vi "1_VisualAD_Train_Eval.vi"(0 "NNFE_Paths":T11={"CFG"=path "D:/Ngene/Projects_SVN/AD/Models/0_Orig/WRN_50_2_1/WRN_50_2_1.cfg", "BIN"=path "D:/Ngene/Projects_SVN/AD/Models/0_Orig/WRN_50_2_1/WRN_50_2_1.bin"}, 1 "Dest. Path":path=path "D:/working/PCB5_append_2025_04_21/21_Data_Leak_Cleaned", 2 "Dataset_Path(Train)":path=path "D:/DNN/_from_Customer/2025_04_11_NIConnect_PCB5/1_Dataset/21_Data_Leak/Train", 3 "Dataset_Path(Validation)":path=path "D:/DNN/_from_Customer/2025_04_11_NIConnect_PCB5/1_Dataset/21_Data_Leak/Test", 4 "Ground_Truth_Folder_Path":path, 5 "error in":errorcluster, 6 "NNFE_CFG":T7={"Name"="PCB5_10K", "Layer_Selection_By"=enum."Stride", "Feature_Layers"={"[LayerID, PatchSize]"=[{"Layer_ID"=8, "Patch_Size"=3}, {"Layer_ID"=16, "Patch_Size"=3}]}, "Interpolation_Type"=enum."Bi-Linear"}, 7 "Dim_Reduction":T5={"Method"=enum."Rnd_Proj", "Target_Dim"=300, "Seed"=42}, 8 "NNPC_Setup":T13={"Input_Dims"={"C"=3, "H"=464, "W"=464}, "mBatch"=1, "Device"=enum."GPU", "GPU Id"=0}, 9 "Coreset_Params":T12={"CoreSet_Size"=10000.0, "Start_idx"=3}) -> (11 "MemBank Size":i32=10000, 13 "dT_Total":dbl=154.27649250000002 format="%.2p", 14 "NNPC_Paths":T11={"CFG"=path "D:/working/PCB5_append_2025_04_21/21_Data_Leak_Cleaned/NNPC_PCB5_10K__25_04_24__18_51_48/NNPC_PCB5_10K.cfg", "BIN"=path "D:/working/PCB5_append_2025_04_21/21_Data_Leak_Cleaned/NNPC_PCB5_10K__25_04_24__18_51_48/NNPC_PCB5_10K.bin"}, 15 "Evaluation_Metrics":T1={"Evaluation_Metrics(Pixel)"={"Scores(Good)"={"X Values"=[0.1535603703558445, 0.16897603914141654, 0.1843917079269886, 0.19980737671256066, 0.2152230454981327, 0.23063871428370475, 0.24605438306927682, 0.26147005185484884, 0.27688572064042094, 0.29230138942599293, 0.30771705821156503, 0.3231327269971371, 0.3385483957827091, 0.35396406456828117, 0.3693797333538532, 0.3847954021394253, 0.4002110709249973, 0.4156267397105694, 0.4310424084961414, 0.4464580772817135, 0.46187374606728554, 0.4772894148528576, 0.4927050836384297, 0.5081207524240017, 0.5235364212095738, 0.5389520899951458, 0.5543677587807179, 0.5697834275662899, 0.585199096351862, 0.6006147651374341, 0.616030433923006, 0.6314461027085781, 0.6468617714941503, 0.6622774402797222, 0.6776931090652942, 0.6931087778508663, 0.7085244466364384, 0.7239401154220104, 0.7393557842075824, 0.7547714529931545, 0.7701871217787266, 0.7856027905642986, 0.8010184593498707, 0.8164341281354428, 0.8318497969210148, 0.8472654657065868, 0.8626811344921589, 0.878096803277731, 0.893512472063303, 0.9089281408488751, 0.9243438096344472, 0.9397594784200192, 0.9551751472055912, 0.9705908159911633, 0.9860064847767354, 1.0014221535623073, 1.0168378223478793, 1.0322534911334516, 1.0476691599190235, 1.0630848287045955, 1.0785004974901677, 1.0939161662757397, 1.1093318350613117, 1.1247475038468837, 1.1401631726324557, 1.155578841418028, 1.1709945102036001, 1.186410178989172, 1.201825847774744, 1.217241516560316, 1.232657185345888, 1.2480728541314603, 1.2634885229170323, 1.2789041917026043, 1.2943198604881765, 1.3097355292737483, 1.3251511980593205, 1.3405668668448927, 1.3559825356304644, 1.3713982044160367, 1.3868138732016086, 1.4022295419871806, 1.4176452107727529, 1.4330608795583248, 1.4484765483438968, 1.463892217129469, 1.4793078859150408, 1.494723554700613, 1.5101392234861852, 1.525554892271757, 1.5409705610573292, 1.5563862298429014, 1.5718018986284732, 1.5872175674140454, 1.6026332361996174, 1.6180489049851894, 1.6334645737707616, 1.6488802425563336, 1.6642959113419056, 1.6797115801274778], "Histogram: h(x)"=[19, 71, 234, 537, 635, 791, 1187, 1664, 4455, 11669, 20450, 27156, 34487, 49909, 89115, 129180, 121277, 93394, 90513, 113616, 128442, 115986, 110386, 119416, 134560, 135091, 138673, 148501, 164573, 180077, 199799, 237706, 287334, 355240, 447708, 578830, 783339, 1110851, 1567027, 2139067, 2671026, 3035938, 3160582, 3051610, 2749404, 2402005, 2090427, 1813597, 1650279, 1570001, 1566516, 1637595, 1767667, 1922699, 2103025, 2248584, 2331421, 2335270, 2221028, 1978020, 1626686, 1226441, 847834, 527127, 293111, 152894, 74763, 33902, 15905, 7259, 3291, 1305, 482, 241, 145, 57, 2, 0, 0, 0, 0, 0, 0, 0, 0, 0, 0, 0, 0, 0, 0, 0, 0, 0, 0, 0, 0, 0, 0, 0]}, "Scores(Bad)"={"X Values"=[0.1535603703558445, 0.16897603914141654, 0.1843917079269886, 0.19980737671256066, 0.2152230454981327, 0.23063871428370475, 0.24605438306927682, 0.26147005185484884, 0.27688572064042094, 0.29230138942599293, 0.30771705821156503, 0.3231327269971371, 0.3385483957827091, 0.35396406456828117, 0.3693797333538532, 0.3847954021394253, 0.4002110709249973, 0.4156267397105694, 0.4310424084961414, 0.4464580772817135, 0.46187374606728554, 0.4772894148528576, 0.4927050836384297, 0.5081207524240017, 0.5235364212095738, 0.5389520899951458, 0.5543677587807179, 0.5697834275662899, 0.585199096351862, 0.6006147651374341, 0.616030433923006, 0.6314461027085781, 0.6468617714941503, 0.6622774402797222, 0.6776931090652942, 0.6931087778508663, 0.7085244466364384, 0.7239401154220104, 0.7393557842075824, 0.7547714529931545, 0.7701871217787266, 0.7856027905642986, 0.8010184593498707, 0.8164341281354428, 0.8318497969210148, 0.8472654657065868, 0.8626811344921589, 0.878096803277731, 0.893512472063303, 0.9089281408488751, 0.9243438096344472, 0.9397594784200192, 0.9551751472055912, 0.9705908159911633, 0.9860064847767354, 1.0014221535623073, 1.0168378223478793, 1.0322534911334516, 1.0476691599190235, 1.0630848287045955, 1.0785004974901677, 1.0939161662757397, 1.1093318350613117, 1.1247475038468837, 1.1401631726324557, 1.155578841418028, 1.1709945102036001, 1.186410178989172, 1.201825847774744, 1.217241516560316, 1.232657185345888, 1.2480728541314603, 1.2634885229170323, 1.2789041917026043, 1.2943198604881765, 1.3097355292737483, 1.3251511980593205, 1.3405668668448927, 1.3559825356304644, 1.3713982044160367, 1.3868138732016086, 1.4022295419871806, 1.4176452107727529, 1.4330608795583248, 1.4484765483438968, 1.463892217129469, 1.4793078859150408, 1.494723554700613, 1.5101392234861852, 1.525554892271757, 1.5409705610573292, 1.5563862298429014, 1.5718018986284732, 1.5872175674140454, 1.6026332361996174, 1.6180489049851894, 1.6334645737707616, 1.6488802425563336, 1.6642959113419056, 1.6797115801274778], "Histogram: h(x)"=[15, 62, 167, 436, 439, 636, 953, 1430, 4212, 9790, 18668, 24642, 27931, 41152, 76605, 105284, 87120, 64040, 68221, 91456, 99939, 85338, 81368, 91950, 104560, 104089, 104569, 115887, 129349, 141297, 162320, 197756, 245867, 310594, 398093, 521655, 715567, 1011400, 1434978, 1933150, 2371176, 2625090, 2582296, 2318639, 1934602, 1521878, 1169314, 929512, 776429, 692764, 672584, 701745, 761058, 844568, 931450, 1018644, 1115656, 1203961, 1254942, 1264724, 1221327, 1119570, 973888, 796667, 632049, 490256, 379906, 296566, 239752, 201233, 178240, 157317, 141343, 130655, 120745, 108950, 97346, 86684, 74229, 61719, 51335, 41546, 34304, 27697, 21602, 18168, 14874, 11980, 8282, 5622, 4047, 3122, 1867, 1094, 601, 280, 136, 86, 64, 34]}, "Eval Stats"={"Scores(Good)"={"Min"=0.14585254, "Max"=1.317711}, "Scores(Bad)"={"Min"=0.15503743, "Max"=1.6874194}, "# of Samples(Good)"=58991104, "# of Samples(Bad)"=43059200, "AUROC"=0.5022648, "F1_Max"=0.5934719, "Thrshld(F1_Max)"=0.1551112, "Prec.(F1_Max)"=0.42194095, "Recall(F1_Max)"=1.0, "FPR(F1_Max)"=0.9999999, "FNR(F1_Max)"=2.322384e-08}}, "Evaluation_Metrics(Image)"={"Scores(Good)"={"X Values"=[1.0789142006635666, 1.0860141378641128, 1.093114075064659, 1.1002140122652053, 1.1073139494657516, 1.1144138866662978, 1.1215138238668443, 1.1286137610673905, 1.1357136982679368, 1.142813635468483, 1.1499135726690293, 1.1570135098695755, 1.1641134470701218, 1.171213384270668, 1.1783133214712143, 1.1854132586717605, 1.1925131958723068, 1.199613133072853, 1.2067130702733992, 1.2138130074739457, 1.220912944674492, 1.2280128818750382, 1.2351128190755845, 1.2422127562761307, 1.249312693476677, 1.2564126306772232, 1.2635125678777694, 1.2706125050783157, 1.277712442278862, 1.2848123794794082, 1.2919123166799544, 1.2990122538805007, 1.3061121910810471, 1.3132121282815934, 1.3203120654821396, 1.3274120026826859, 1.3345119398832321, 1.3416118770837784, 1.3487118142843246, 1.3558117514848709, 1.3629116886854171, 1.3700116258859634, 1.3771115630865096, 1.3842115002870559, 1.3913114374876023, 1.3984113746881486, 1.4055113118886948, 1.412611249089241, 1.4197111862897873, 1.4268111234903336, 1.4339110606908798, 1.441010997891426, 1.4481109350919723, 1.4552108722925186, 1.4623108094930648, 1.469410746693611, 1.4765106838941573, 1.4836106210947035, 1.4907105582952498, 1.4978104954957963, 1.5049104326963425, 1.5120103698968888, 1.519110307097435, 1.5262102442979812, 1.5333101814985275, 1.5404101186990737, 1.54751005589962, 1.5546099931001662, 1.5617099303007125, 1.568809867501259, 1.5759098047018052, 1.5830097419023514, 1.5901096791028977, 1.597209616303444, 1.6043095535039902, 1.6114094907045364, 1.6185094279050827, 1.625609365105629, 1.6327093023061752, 1.6398092395067214, 1.6469091767072677, 1.654009113907814, 1.6611090511083602, 1.6682089883089064, 1.6753089255094527, 1.682408862709999, 1.6895087999105454, 1.6966087371110916, 1.7037086743116379, 1.710808611512184, 1.7179085487127304, 1.7250084859132766, 1.7321084231138228, 1.7392083603143693, 1.7463082975149156, 1.7534082347154618, 1.760508171916008, 1.7676081091165543, 1.7747080463171006, 1.7818079835176468], "Histogram: h(x)"=[1, 0, 0, 0, 0, 0, 0, 0, 0, 0, 0, 1, 0, 0, 0, 0, 1, 2, 2, 4, 7, 21, 16, 24, 30, 12, 19, 17, 23, 18, 11, 7, 9, 7, 14, 6, 2, 6, 5, 1, 3, 0, 0, 1, 1, 1, 0, 1, 0, 1, 0, 0, 0, 0, 0, 0, 0, 0, 0, 0, 0, 0, 0, 0, 0, 0, 0, 0, 0, 0, 0, 0, 0, 0, 0, 0, 0, 0, 0, 0, 0, 0, 0, 0, 0, 0, 0, 0, 0, 0, 0, 0, 0, 0, 0, 0, 0, 0, 0, 0]}, "Scores(Bad)"={"X Values"=[1.0789142006635666, 1.0860141378641128, 1.093114075064659, 1.1002140122652053, 1.1073139494657516, 1.1144138866662978, 1.1215138238668443, 1.1286137610673905, 1.1357136982679368, 1.142813635468483, 1.1499135726690293, 1.1570135098695755, 1.1641134470701218, 1.171213384270668, 1.1783133214712143, 1.1854132586717605, 1.1925131958723068, 1.199613133072853, 1.2067130702733992, 1.2138130074739457, 1.220912944674492, 1.2280128818750382, 1.2351128190755845, 1.2422127562761307, 1.249312693476677, 1.2564126306772232, 1.2635125678777694, 1.2706125050783157, 1.277712442278862, 1.2848123794794082, 1.2919123166799544, 1.2990122538805007, 1.3061121910810471, 1.3132121282815934, 1.3203120654821396, 1.3274120026826859, 1.3345119398832321, 1.3416118770837784, 1.3487118142843246, 1.3558117514848709, 1.3629116886854171, 1.3700116258859634, 1.3771115630865096, 1.3842115002870559, 1.3913114374876023, 1.3984113746881486, 1.4055113118886948, 1.412611249089241, 1.4197111862897873, 1.4268111234903336, 1.4339110606908798, 1.441010997891426, 1.4481109350919723, 1.4552108722925186, 1.4623108094930648, 1.469410746693611, 1.4765106838941573, 1.4836106210947035, 1.4907105582952498, 1.4978104954957963, 1.5049104326963425, 1.5120103698968888, 1.519110307097435, 1.5262102442979812, 1.5333101814985275, 1.5404101186990737, 1.54751005589962, 1.5546099931001662, 1.5617099303007125, 1.568809867501259, 1.5759098047018052, 1.5830097419023514, 1.5901096791028977, 1.597209616303444, 1.6043095535039902, 1.6114094907045364, 1.6185094279050827, 1.625609365105629, 1.6327093023061752, 1.6398092395067214, 1.6469091767072677, 1.654009113907814, 1.6611090511083602, 1.6682089883089064, 1.6753089255094527, 1.682408862709999, 1.6895087999105454, 1.6966087371110916, 1.7037086743116379, 1.710808611512184, 1.7179085487127304, 1.7250084859132766, 1.7321084231138228, 1.7392083603143693, 1.7463082975149156, 1.7534082347154618, 1.760508171916008, 1.7676081091165543, 1.7747080463171006, 1.7818079835176468], "Histogram: h(x)"=[0, 0, 0, 0, 0, 0, 0, 0, 0, 0, 0, 0, 0, 0, 0, 0, 0, 0, 0, 0, 0, 0, 0, 0, 0, 0, 0, 0, 0, 0, 0, 0, 0, 0, 0, 0, 0, 0, 0, 0, 0, 0, 0, 0, 0, 0, 0, 0, 0, 0, 0, 0, 0, 1, 0, 0, 1, 1, 2, 1, 6, 1, 3, 10, 5, 5, 7, 5, 15, 17, 9, 11, 13, 7, 10, 10, 8, 7, 6, 4, 7, 5, 7, 3, 4, 3, 3, 1, 0, 1, 0, 0, 0, 0, 0, 0, 0, 0, 0, 1]}, "Eval Stats"={"Scores(Good)"={"Min"=1.0753642, "Max"=1.4269079}, "Scores(Bad)"={"Min"=1.4559232, "Max"=1.785358}, "# of Samples(Good)"=274, "# of Samples(Bad)"=200, "AUROC"=1.0, "F1_Max"=1.0, "Thrshld(F1_Max)"=1.4414155, "Prec.(F1_Max)"=1.0, "Recall(F1_Max)"=1.0, "FPR(F1_Max)"=0.0, "FNR(F1_Max)"=0.0}}} {"Evaluation_Metrics(Image)"."Eval Stats"."Recall(F1_Max)" format="%#.5f"; "Evaluation_Metrics(Image)"."Eval Stats"."FPR(F1_Max)" format="%#.5f"; "Evaluation_Metrics(Image)"."Eval Stats"."FNR(F1_Max)" format="%#.5f"; "Evaluation_Metrics(Image)"."Eval Stats"."Prec.(F1_Max)" format="%#.5f"; "Evaluation_Metrics(Image)"."Eval Stats"."F1_Max" format="%#.5f"; "Evaluation_Metrics(Image)"."Eval Stats"."AUROC" format="%#.5f"; "Evaluation_Metrics(Image)"."Eval Stats"."Scores(Bad)"."Min" format="%#_5g"; "Evaluation_Metrics(Image)"."Eval Stats"."Scores(Good)"."Min" format="%#_5g"; "Evaluation_Metrics(Image)"."Eval Stats"."Thrshld(F1_Max)" format="%#_5f"; "Evaluation_Metrics(Pixel)"."Eval Stats"."Recall(F1_Max)" format="%#.5f"; "Evaluation_Metrics(Pixel)"."Eval Stats"."FPR(F1_Max)" format="%#.5f"; "Evaluation_Metrics(Pixel)"."Eval Stats"."FNR(F1_Max)" format="%#.5f"; "Evaluation_Metrics(Pixel)"."Eval Stats"."Prec.(F1_Max)" format="%#.5f"; "Evaluation_Metrics(Pixel)"."Eval Stats"."F1_Max" format="%#.5f"; "Evaluation_Metrics(Pixel)"."Eval Stats"."AUROC" format="%#.5f"; "Evaluation_Metrics(Pixel)"."Eval Stats"."Scores(Bad)"."Min" format="%#_5g"; "Evaluation_Metrics(Pixel)"."Eval Stats"."Scores(Good)"."Min" format="%#_5g"; "Evaluation_Metrics(Pixel)"."Eval Stats"."Thrshld(F1_Max)" format="%#_5f"}, 18 "Dataset Size":i32=1056)   [LabVIEW 2020]
uses:
  <vilib>/Ngene/DeepLTK Anomaly Detection Addon/DeepLTK_Anomaly_Detection_Addon/API/Controls/NN_Paths.ctl
  <vilib>/Ngene/DeepLTK Anomaly Detection Addon/DeepLTK_Anomaly_Detection_Addon/API/Controls/NNPC_Setup.ctl
  <vilib>/Ngene/Deep Learning Toolkit/Toolkit/NN_Data/API/NN_Dims(C,H,W).ctl
  <vilib>/Ngene/Deep Learning Toolkit/Toolkit/NN_Network/Controls/NN_Device.ctl
  <vilib>/Ngene/DeepLTK Anomaly Detection Addon/DeepLTK_Anomaly_Detection_Addon/API/Controls/NNPC_Coreset_Params.ctl
  <vilib>/Ngene/DeepLTK Anomaly Detection Addon/DeepLTK_Anomaly_Detection_Addon/API/Controls/NNFE_CFG.ctl
  <vilib>/Ngene/DeepLTK Anomaly Detection Addon/DeepLTK_Anomaly_Detection_Addon/API/Controls/Layer_Selector.ctl
  <vilib>/Ngene/DeepLTK Anomaly Detection Addon/DeepLTK_Anomaly_Detection_Addon/API/Controls/Feature_Layer_Selector.ctl
  <vilib>/Ngene/DeepLTK Anomaly Detection Addon/DeepLTK_Anomaly_Detection_Addon/API/Controls/Interpolation_Selector.ctl
  <vilib>/Ngene/DeepLTK Anomaly Detection Addon/DeepLTK_Anomaly_Detection_Addon/API/Controls/NNPC_Random_Projection_CFG.ctl
  <vilib>/Ngene/DeepLTK Anomaly Detection Addon/DeepLTK_Anomaly_Detection_Addon/API/Controls/Dim_Reduction_Method.ctl
  <vilib>/Ngene/DeepLTK Anomaly Detection Addon/DeepLTK_Anomaly_Detection_Addon/API/Controls/Evaluation_Metrics(Pixel_Image).ctl
  <vilib>/Ngene/DeepLTK Anomaly Detection Addon/DeepLTK_Anomaly_Detection_Addon/API/Controls/Evaluation_Metrics.ctl
  <vilib>/Ngene/DeepLTK Anomaly Detection Addon/DeepLTK_Anomaly_Detection_Addon/API/Controls/Eval_Results.ctl
  <vilib>/Ngene/DeepLTK Anomaly Detection Addon/DeepLTK_Anomaly_Detection_Addon/API/Controls/MinMax.ctl
  <vilib>/Ngene/DeepLTK Anomaly Detection Addon/DeepLTK_Anomaly_Detection_Addon/API/Controls/Feature_Scorer_Params.ctl
  <vilib>/Ngene/DeepLTK Anomaly Detection Addon/DeepLTK_Anomaly_Detection_Addon/API/Controls/Gaussian_Blur.ctl
  <vilib>/Ngene/DeepLTK Anomaly Detection Addon/DeepLTK_Anomaly_Detection_Addon/API/Controls/NNPC_Save_CFG.ctl
  <vilib>/Ngene/DeepLTK Anomaly Detection Addon/DeepLTK_Anomaly_Detection_Addon/API/Controls/NNPC_PreProcessing_Options.ctl
  <vilib>/Ngene/DeepLTK Anomaly Detection Addon/DeepLTK_Anomaly_Detection_Addon/API/Controls/NNPC_DS_Stats.ctl
  <vilib>/Ngene/DeepLTK Anomaly Detection Addon/DeepLTK_Anomaly_Detection_Addon/API/Controls/Image_Stats_RGB.ctl
  subVIs/Dataset_Reader/Controls/Read_Options.ctl
  <vilib>/Ngene/DeepLTK Anomaly Detection Addon/DeepLTK_Anomaly_Detection_Addon/API/NNPC_Generate_Embedding/NNPC_Generate_Embedding(Dataset).vi
  <vilib>/Ngene/DeepLTK Anomaly Detection Addon/DeepLTK_Anomaly_Detection_Addon/API/NNPC_Predict/NNPC_Predict(Dataset).vi
  <vilib>/Ngene/Deep Learning Toolkit/Toolkit/NN_Data/subVIs/Dataset_Destroy/NN_Dataset_Destroy(In3D_Out3D).vi
  <vilib>/Ngene/Deep Learning Toolkit/Toolkit/Deep_Learning_Toolkit_by_Ngene.lvlib
  <vilib>/Ngene/DeepLTK Anomaly Detection Addon/DeepLTK_Anomaly_Detection_Addon/DeepLTK_Anomaly_Detection_Addon.lvlib
panel:
  out "Feature Size":i32=300
  out "error out":errorcluster
  out "Coreset Min":sgl=1.2493105
  out "Coreset Max":sgl=3.675024
  out "dT_Predict":dbl=7.602655700000014 format="%.2p"
  out "dT_Eval":dbl=30.186260299999958 format="%.2p"
  out "dT_Read_DS(Test)":dbl=6.505981099999985 format="%.2p"
  out "dT_Read_DS(Train)":dbl=17.761814999999956 format="%.2p"
  out "dT_NN_Init":dbl=6.9475914000000785 format="%.2p"
  out "Coreset_Max_Distances":sgl[](graph)
  out "dT_Coreset":dbl=85.95763010000007 format="%.2p"
  out "dT_Gen_Embed":dbl=12.12111630000004 format="%.2p"
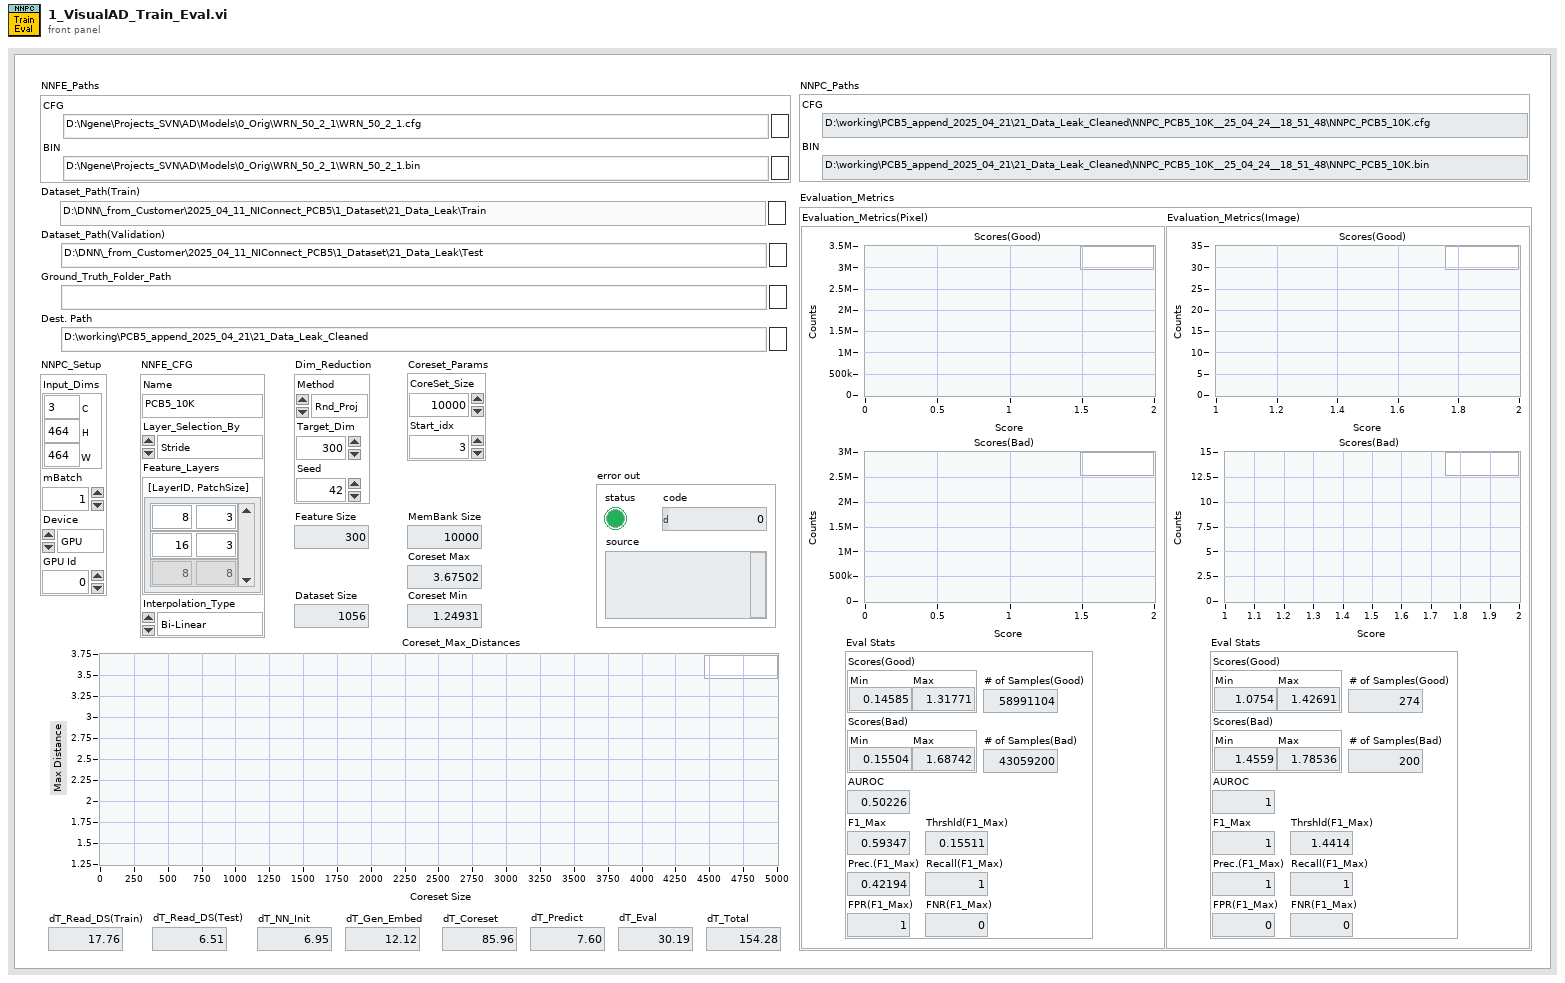
[diagram p1: front panel]
types:
  T1 = typedef "DeepLTK_Anomaly_Detection_Addon.lvlib/Evaluation_Metrics(Pixel_Image).ctl" = cluster{"Evaluation_Metrics(Pixel)":T2, "Evaluation_Metrics(Image)":T2}
  T2 = typedef "DeepLTK_Anomaly_Detection_Addon.lvlib/Evaluation_Metrics.ctl" = cluster{"Scores(Good)":cluster{"X Values":dbl[], "Histogram: h(x)":i32[]}, "Scores(Bad)":cluster{"X Values":dbl[], "Histogram: h(x)":i32[]}, "Eval Stats":T3}
  T3 = typedef "DeepLTK_Anomaly_Detection_Addon.lvlib/Eval_Results.ctl" = cluster{"Scores(Good)":T4, "Scores(Bad)":T4, "# of Samples(Good)":i32, "# of Samples(Bad)":i32, "AUROC":sgl, "F1_Max":sgl, "Thrshld(F1_Max)":sgl, "Prec.(F1_Max)":sgl, "Recall(F1_Max)":sgl, "FPR(F1_Max)":sgl, "FNR(F1_Max)":sgl}
  T4 = typedef "DeepLTK_Anomaly_Detection_Addon.lvlib/MinMax.ctl" = cluster{"Min":sgl, "Max":sgl}
  T5 = typedef "DeepLTK_Anomaly_Detection_Addon.lvlib/NNPC_Random_Projection_CFG.ctl" = cluster{"Method":T6, "Target_Dim":i32, "Seed":i32}
  T6 = typedef "DeepLTK_Anomaly_Detection_Addon.lvlib/Dim_Reduction_Method.ctl" = enum16{"None", "Rnd_Proj", "PCA"}
  T7 = typedef "DeepLTK_Anomaly_Detection_Addon.lvlib/NNFE_CFG.ctl" = cluster{"Name":string, "Layer_Selection_By":T8, "Feature_Layers":T9, "Interpolation_Type":T10}
  T8 = typedef "DeepLTK_Anomaly_Detection_Addon.lvlib/Layer_Selector.ctl" = enum16{"Stride", "Layer_Idx"}
  T9 = typedef "DeepLTK_Anomaly_Detection_Addon.lvlib/Feature_Layer_Selector.ctl" = cluster{"[LayerID, PatchSize]":cluster{"Layer_ID":i32, "Patch_Size":i32}[]}
  T10 = typedef "DeepLTK_Anomaly_Detection_Addon.lvlib/Interpolation_Selector.ctl" = enum16{"Nearest", "Bi-Linear"}
  T11 = typedef "DeepLTK_Anomaly_Detection_Addon.lvlib/NN_Paths.ctl" = cluster{"CFG":path, "BIN":path}
  T12 = typedef "DeepLTK_Anomaly_Detection_Addon.lvlib/NNPC_Coreset_Params.ctl" = cluster{"CoreSet_Size":sgl, "Start_idx":i32}
  T13 = typedef "DeepLTK_Anomaly_Detection_Addon.lvlib/NNPC_Setup.ctl" = cluster{"Input_Dims":T14, "mBatch":i32, "Device":T15, "GPU Id":i32}
  T14 = typedef "Deep_Learning_Toolkit_by_Ngene.lvlib/NN_Dims(C,H,W).ctl" = cluster{"C":i32, "H":i32, "W":i32}
  T15 = typedef "Deep_Learning_Toolkit_by_Ngene.lvlib/NN_Device.ctl" = enum16{"CPU", "GPU"}
  T16 = typedef "DeepLTK_Anomaly_Detection_Addon.lvlib/Feature_Scorer_Params.ctl" = cluster{"Nearest_Neighbors":i32, "Calculate Anomaly Map":bool, "Gaussian_Blur":T17}
  T17 = typedef "DeepLTK_Anomaly_Detection_Addon.lvlib/Gaussian_Blur.ctl" = cluster{"Kernel_Size":i32, "Sigma":sgl}
  T18 = typedef "DeepLTK_Anomaly_Detection_Addon.lvlib/NNPC_Save_CFG.ctl" = cluster{"Add_TimeStamp_SubFolder":bool, "Append_TimeStamp_to_FileNames":bool}
  T19 = typedef "DeepLTK_Anomaly_Detection_Addon.lvlib/NNPC_PreProcessing_Options.ctl" = cluster{"DS_Name":string, "Input_Dims":T14, "Center Crop Size":i32, "Interpolation Type":u32, "Multi-Stage_DownSample?":bool, "Dataset_Stats":T20}
  T20 = typedef "DeepLTK_Anomaly_Detection_Addon.lvlib/NNPC_DS_Stats.ctl" = cluster{"means":T21, "stds":T21}
  T21 = typedef "DeepLTK_Anomaly_Detection_Addon.lvlib/Image_Stats_RGB.ctl" = cluster{"R":sgl, "G":sgl, "B":sgl}
  T22 = typedef "Read_Options.ctl" = cluster{"Read Bads?":bool, "Read GTs?":bool, "Update. DS Stats?":bool}
  T23 = typedef "Deep_Learning_Toolkit_by_Ngene.lvlib/NN_DataSet(In3D_Out3D).ctl" = cluster{"Dataset_Size":i32, "Dims_In":T14, "Labels":string[], "File Paths":path[], "Outputs Ref.":T24, "Inputs Ref.":variant, "Dims_Out":T14}
  T24 = typedef "Deep_Learning_Toolkit_by_Ngene.lvlib/NN_Data_ref(4D_SGL).ctl" = refnum<data-value>
  T25 = typedef "DeepLTK_Anomaly_Detection_Addon.lvlib/NNPC_Instance.ctl" = cluster{"NN":T26, "MemBank_Data":T41, "Name":string}
  T26 = typedef "Deep_Learning_Toolkit_by_Ngene.lvlib/NN.ctl" = cluster{"Name":string, "No of Layers":i32, "mBatch":i32, "Layers":T27[], "Dimty":T28, "Dims_In":T14, "Dims_Out":T14, "Working_Dir":path, "Train?":bool, "Train_Params":T29, "LR_Update_Policy":T32, "Session Data":T34, "Ground_truth":T35, "NNg_hdls":T36, "NN_Device":T15, "GPU Id":i32, "Labels":string[], "Receptive Field":T37[], "Loss_Type":T38, "Loss_Cfg_Prms":variant, "NNG_WS":T39}
  T27 = typedef "Deep_Learning_Toolkit_by_Ngene.lvlib/NN_Layer_ref.ctl" = refnum<data-value>
  T28 = typedef "Deep_Learning_Toolkit_by_Ngene.lvlib/NN_In_Out_Dim-ty.ctl" = enum8{"In1D_Out1D", "In3D_Out1D", "In3D_Out3D", "In3D_OutBBox"}
  T29 = typedef "Deep_Learning_Toolkit_by_Ngene.lvlib/NN_Train_Params.ctl" = cluster{"Optimizer":T30, "Beta_1":sgl, "Beta_2":sgl, "Weight Decay(L1)":sgl, "Weight Decay(L2)":sgl, "Data_Sampling":T31}
  T30 = typedef "Deep_Learning_Toolkit_by_Ngene.lvlib/NN_Train_Optimizer.ctl" = enum16{"SGD", "Adam", "Adagrad", "Adadelta", "RMSProp", "Nesterov"}
  T31 = typedef "Deep_Learning_Toolkit_by_Ngene.lvlib/NN_Train_Data_Sampling.ctl" = enum16{"Random", "Sequential"}
  T32 = typedef "Deep_Learning_Toolkit_by_Ngene.lvlib/NN_LR_Policy_Cfg.ctl" = cluster{"Policy_Type":T33, "LR0":dbl, "k":sgl, "WarmUp_Policy":enum16{"Step", "Ramp"}, "WarmUp_Iter":i32, "WarmUp_Ratio":sgl}
  T33 = typedef "Deep_Learning_Toolkit_by_Ngene.lvlib/NN_LR_Policy_Type.ctl" = enum16{"Manual", "Step", "Exp", "1/t"}
  T34 = typedef "Deep_Learning_Toolkit_by_Ngene.lvlib/NN_Train_Session_Data.ctl" = cluster{"Epochs":sgl, "Tot_Iter":i32, "LR":sgl, "LR_iter":i32}
  T35 = typedef "Deep_Learning_Toolkit_by_Ngene.lvlib/NN_Ground_truth.ctl" = cluster{"Y":variant}
  T36 = typedef "Deep_Learning_Toolkit_by_Ngene.lvlib/nng_cuda_handles.ctl" = cluster{"cudnn":u64, "cublas":u64, "stream":u64, "curand":u64}
  T37 = typedef "Deep_Learning_Toolkit_by_Ngene.lvlib/NN_Dims(V,H).ctl" = cluster{"V":i32, "H":i32}
  T38 = typedef "Deep_Learning_Toolkit_by_Ngene.lvlib/NN_Loss_Type.ctl" = enum16{"None", "MSE", "CrossEntropy", "YOLO_v2", "YOLO_v4"}
  T39 = typedef "Deep_Learning_Toolkit_by_Ngene.lvlib/NNG_WS.ctl" = cluster{"NNG_WS_Mem":T40, "Max_WS_Size":i64}
  T40 = typedef "Deep_Learning_Toolkit_by_Ngene.lvlib/NNg_WS_Mem_DVR.ctl" = refnum<data-value>
  T41 = typedef "DeepLTK_Anomaly_Detection_Addon.lvlib/MemBank_and_Norm_Variants.ctl" = cluster{"MemBank":variant, "MemBank Norm":variant}
  T42 = typedef "imagedata.ctl" = cluster{"image type":i32, "image depth":i32, "image":u8[], "mask":u8[], "colors":u32[], "Rectangle":cluster{"left":i16, "top":i16, "right":i16, "bottom":i16}}
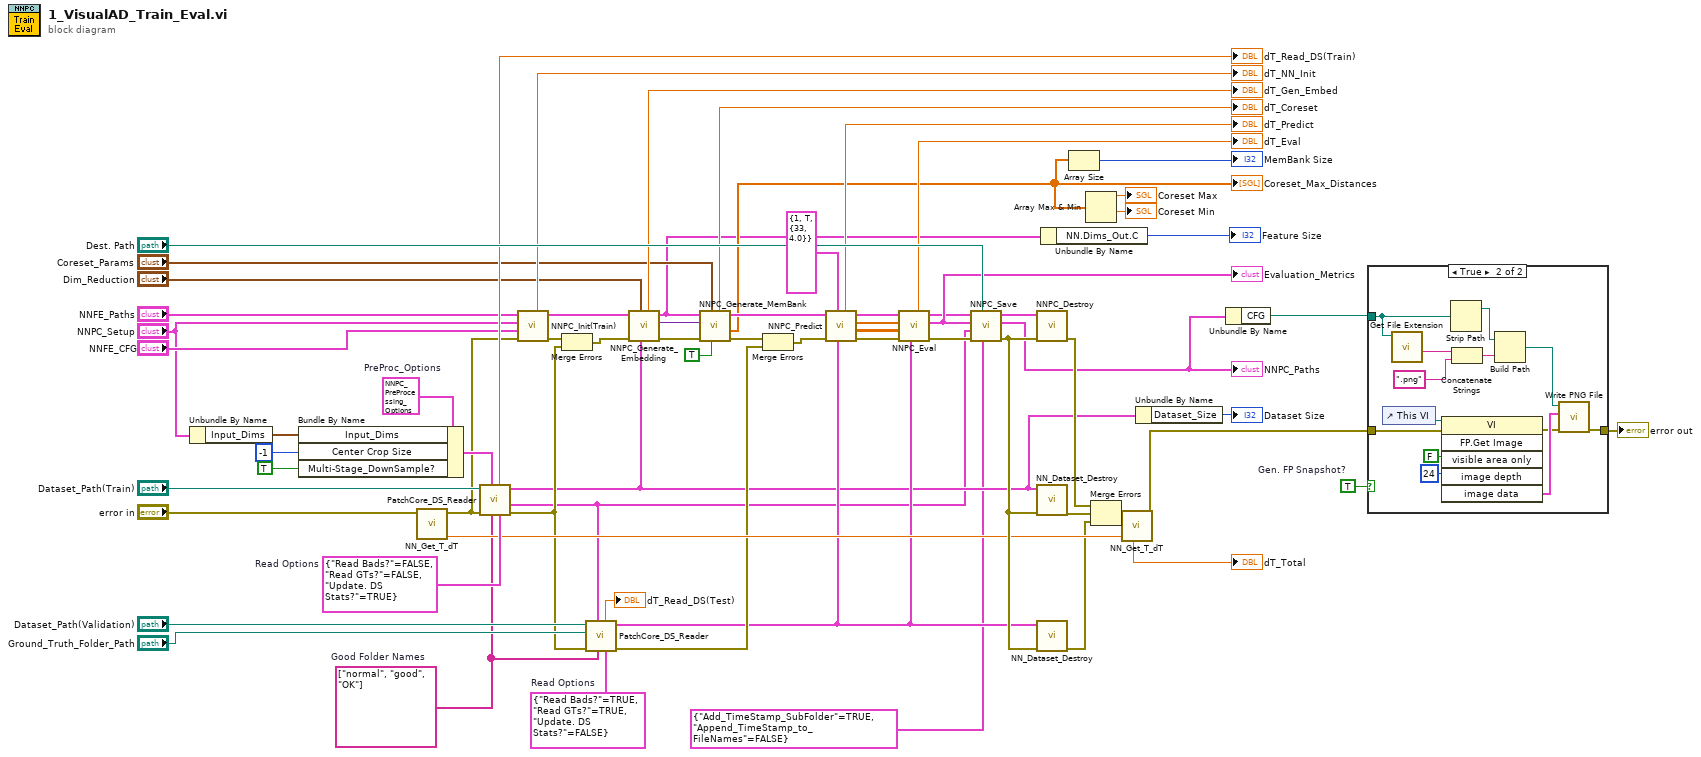
[diagram p0: block diagram]
diagram:
  w5 = T19 {"DS_Name"="", "Input_Dims"={"C"=3, "H"=224, "W"=224}, "Center Crop Size"=0, "Interpolation Type"=1, "Multi-Stage_DownSample?"=FALSE, "Dataset_Stats"={"means"={"R"=0.0, "G"=0.0, "B"=0.0}, "stds"={"R"=1.0, "G"=1.0, "B"=1.0}}}  # PreProc_Options
  w22 = TRUE  # Gen. FP Snapshot?
  w50 = T22 {"Read Bads?"=TRUE, "Read GTs?"=TRUE, "Update. DS Stats?"=FALSE}  # Read Options
  w56 = T22 {"Read Bads?"=FALSE, "Read GTs?"=FALSE, "Update. DS Stats?"=TRUE}  # Read Options
  w32 = string[] ["normal", "good", "OK"]  # Good Folder Names
  n1 = Unbundle By Name("NNPC_Setup") -> ("Input_Dims"=w57:T14)
  n2 = Bundle By Name(cluster=w5, "Input_Dims"=w57, "Center Crop Size"=-1, "Multi-Stage_DownSample?"=TRUE) -> (w24:T19)
  n3 = call <vilib>:"NN_Get_T_dT.vi"("error in (no error)"="error in") -> ("T_out"=w54:dbl, "error out"=w13:errorcluster)  [unwired: 6 in, 1 out]
  n4 = call "PatchCore_DS_Reader.vi"("Read Options"=w56, "Good Unique Labels"=w32, "PreProc_Options_in"=w24, "error in (no error)"=w13, "Folder Path"="Dataset_Path(Train)") -> ("error out"=w46:errorcluster, "PreProc_Options_out"=w4:T19, "Dataset"=w25:T23, "dT_DS_Reader"=→"dT_Read_DS(Train)":dbl)  [unwired: 3 in]
  n5 = call <vilib>:"NNPC_Init(Train).vi"("error in"=w13, "NNFE_CFG"="NNFE_CFG", "NNPC_Setup"="NNPC_Setup", "NNFE_Paths"="NNFE_Paths") -> ("error out"=w63:errorcluster, "NNPC_out"=w62:T25, "dT_Init_Train"=→"dT_NN_Init":dbl)  [unwired: 5 in]
  n6 = Merge Errors(w63, w46) -> (w15:errorcluster)
  n7 = call "PatchCore_DS_Reader.vi"("Read Options"=w50, "Good Unique Labels"=w32, "PreProc_Options_in"=w4, "error in (no error)"=w46, "GT Folder Path"="Ground_Truth_Folder_Path", "Folder Path"="Dataset_Path(Validation)") -> ("error out"=w37:errorcluster, "Dataset"=w36:T23, "dT_DS_Reader"=→"dT_Read_DS(Test)":dbl)  [unwired: 2 in, 1 out]
  n8 = call-poly <vilib>:"NNPC_Generate_Embedding.vi"("Dataset"=w25, "Dim_Reduction"="Dim_Reduction", "error in"=w15, "NNPC_in"=w62) -> ("error out"=w14:errorcluster, "Feature_Embeddings"=w16:variant, "NNPC_out"=w7:T25, "dT_Embed"=→"dT_Gen_Embed":dbl)  [unwired: 3 in, 1 out]
  n9 = call <vilib>:"NNPC_Generate_MemBank.vi"("Destroy Embeds Afterwards?"=TRUE, "Coreset_Params"="Coreset_Params", "error in (no error)"=w14, "Feature_Embeddings"=w16, "NNPC_in"=w7) -> ("error out"=w23:errorcluster, "Max_Distances"=w12:sgl[], "NNPC_out"=w40:T25, "dT_Coreset"=→"dT_Coreset":dbl)  [unwired: 3 in]
  "Coreset_Max_Distances" <- w12
  n10 = Merge Errors(w23, w37) -> (w38:errorcluster)
  n11 = call-poly <vilib>:"NNPC_Predict.vi"("Dataset"=w36, "Feature_Scorer_Params"=T16 {"Nearest_Neighbors"=1, "Calculate Anomaly Map"=TRUE, "Gaussian_Blur"={"Kernel_Size"=33, "Sigma"=4.0}}, "error in (no error)"=w38, "NNPC_in"=w40) -> ("error out"=w41:errorcluster, "Anomaly_Maps"=w43:sgl[][][], "Pred_Scores"=w44:sgl[], "NNPC_out"=w30:T25, "dT_Predict"=→"dT_Predict":dbl)  [unwired: 3 in]
  n12 = call <vilib>:"NNPC_Eval.vi"("Dataset"=w36, "error in (no error)"=w41, "Anomaly_Maps"=w43, "Pred_Scores"=w44, "NNPC_in"=w30) -> ("error out"=w39:errorcluster, "Evaluation_Metrics"=w31:T1, "NNPC_out"=w29:T25, "dT_Eval"=→"dT_Eval":dbl)  [unwired: 3 in]
  "Evaluation_Metrics" <- w31
  n13 = call <vilib>:"NNPC_Save.vi"("Save_Config"=T18 {"Add_TimeStamp_SubFolder"=TRUE, "Append_TimeStamp_to_FileNames"=FALSE}, "Dst_Folder"="Dest. Path", "error in (no error)"=w39, "PreProc_Options_in"=w4, "Evaluation Metrics"=w31, "NNPC_in"=w29) -> ("error out"=w69:errorcluster, "NNPC_Paths"=w21:T11, "NNPC_out"=w8:T25)  [unwired: 3 in]
  "NNPC_Paths" <- w21
  n14 = call <vilib>:"NNPC_Destroy.vi"("error in"=w69, "NNPC_in"=w8) -> ("error out"=w67:errorcluster)  [unwired: 9 in]
  n15 = call-poly <vilib>:"NN_Dataset_Destroy.vi"("error in (no error)"=w69, "Dataset(In3D_Out3D)"=w25) -> ("error out"=w34:errorcluster)  [unwired: 9 in]
  n16 = call-poly <vilib>:"NN_Dataset_Destroy.vi"("error in (no error)"=w69, "Dataset(In3D_Out3D)"=w36) -> ("error out"=w33:errorcluster)  [unwired: 9 in]
  n17 = Unbundle By Name(w7) -> ("NN.Dims_Out.C"=→"Feature Size":i32)
  n18 = Array Size(array=w12) -> (size(s)=→"MemBank Size":i32)
  n19 = Array Max & Min(array=w12) -> (max value=→"Coreset Max":sgl, min value=→"Coreset Min":sgl)  [unwired: 2 out]
  n20 = Merge Errors(w67, w34, w33) -> (w35:errorcluster)
  n21 = call <vilib>:"NN_Get_T_dT.vi"("T_in"=w54, "error in (no error)"=w35) -> ("error out"=w17:errorcluster, "dT"=→"dT_Total":dbl)  [unwired: 5 in, 1 out]
  n22 = Unbundle By Name(w25) -> ("Dataset_Size"=→"Dataset Size":i32)
  n23 = Unbundle By Name(w21) -> ("CFG"=w20:path)
  n24 = case shown="True" w22 {
    tunnel: w20 -> [_ w73]
    tunnel: w17 -> [w70 w72]
    tunnel: [w70 w71] -> w9
    frame False {
    }
    frame True {
      n25 = control-ref of="This VI"() -> (w83:refnum<vi>)
      n26 = call <vilib>:"Get File Extension.vi"("file"=w73) -> ("filename without extension"=w78:string)  [unwired: 6 in, 4 out]
      n27 = invoke class="VI" method="FP.Get Image"(reference=w83, error in=w72, "visible area only"=FALSE ("Visible Area Only"), "image depth"=24 ("Image Depth")) -> (error out=w79:errorcluster, "image data"=w80:T42)  [unwired: 2 in, 4 out]
      n28 = Strip Path(path=w73) -> (stripped path=w75:path)  [unwired: 1 out]
      n29 = Concatenate Strings(w78, ".png" ("string")) -> (w76:string)
      n30 = Build Path(base path=w75, name or relative path=w76) -> (appended path=w74:path)
      n31 = call <vilib>:"Write PNG File.vi"("error in (no error)"=w79, "image data"=w80, "path to PNG file"=w74) -> ("error out"=w71:errorcluster)  [unwired: 7 in, 1 out]
    }
  }
  "error out" <- w9
